vi "test_ExposureTimeJsonSet.vi"   [LabVIEW 2023]
uses:
  23d85119-80bc-4272-b841-6b19ecefd2d9.vi
  <vilib>/JDP Science/JSONtext/Variant to JSON Text.vi
  <vilib>/JDP Science/JSONtext/Set Item.vi
  <vilib>/addons/_JKI Toolkits/Caraya/classes/Assert/Assert Equal Value and Type_Variant.vi
  <vilib>/JDP Science/JSONtext/LVClass Serializer/JSONtext LVClass Serializer.lvclass
  <vilib>/addons/_JKI Toolkits/Caraya/classes/Test/Test.lvclass
  <vilib>/addons/_JKI Toolkits/Caraya/classes/Assert/Assert.lvclass
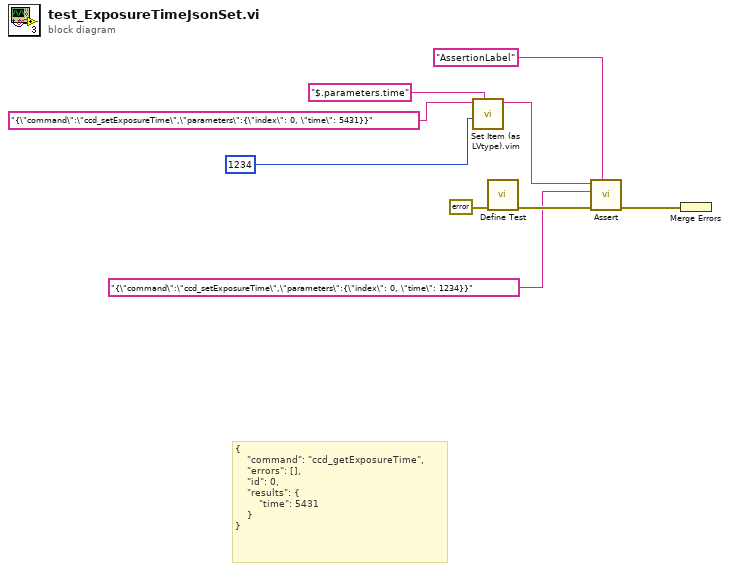
[diagram p0: block diagram]
diagram:
  # "{\n    \"command\": \"ccd_getExposureTime\",\n    \"errors\": [],\n    \"id\": 0,\n    \"results\": {\n        \"time\": 5431\n    }\n}"
  n1 = call "Set Item (as LVtype).vim"("$Path or Item Name"="$.parameters.time", "Anything"=1234, "JSON"="{\"command\":\"ccd_setExposureTime\",\"parameters\":{\"index\": 0, \"time\": 5431}}") -> ("<JSON>"=w2:string)  [unwired: 5 in, 2 out]
  n2 = call <vilib>:"Define Test.vi"("error in (no error)"=errorcluster {"status"=FALSE, "code"=0, "source"=""}) -> ("error out"=w7:errorcluster)  [unwired: 9 in, 1 out]
  n3 = call-poly <vilib>:"Assert.vi"("Label"="AssertionLabel" ("Label (VI Title)"), "error in (no error)"=w7, "Y"="{\"command\":\"ccd_setExposureTime\",\"parameters\":{\"index\": 0, \"time\": 1234}}", "X"=w2) -> ("error out"=w8:errorcluster)  [unwired: 6 in, 1 out]
  n4 = Merge Errors(w8) -> ()  [unwired: 1 out]
